vi "Add New Data Channels.vi"(8 "error in (no error)":errorcluster, 11 "Node Ptr":u64 format="%.0x") -> (0 "error out":errorcluster)   [LabVIEW 2019]
uses:
  <vilib>/NI VeriStand/Custom Device API/Custom Device Channel.ctl
  <vilib>/NI VeriStand/Custom Device API/Custom Device Channel Type.ctl
  Shared/Constants.vi
  <vilib>/NI VeriStand/Custom Device API/Set Item Property (String).vi
  <vilib>/NI VeriStand/Custom Device API/Custom Device API.lvlib
  Shared/Instrument Addon Shared.lvlib
panel:
  in  "Tag":string
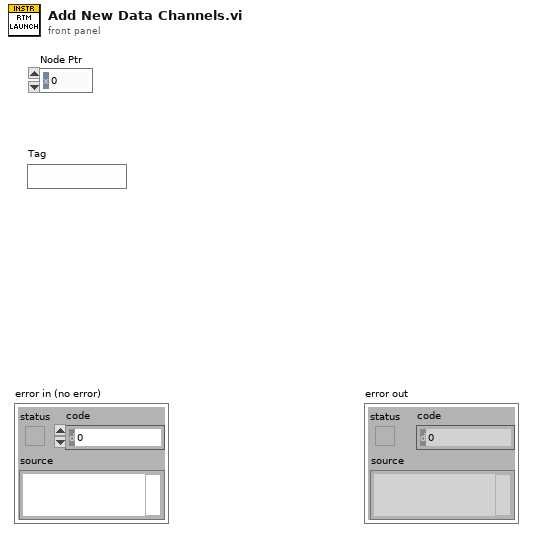
[diagram p1: front panel]
types:
  T1 = typedef "Custom Device API.lvlib/Custom Device Channel.ctl" = cluster{"Type":T2, "Units":string, "Default Value":dbl, "Faultable":bool, "Scalable":bool}
  T2 = typedef "Custom Device API.lvlib/Custom Device Channel Type.ctl" = enum16{"Input", "Output"}
  T3 = typedef "Custom Device API.lvlib/Custom Device Item Ref.ctl" = u64
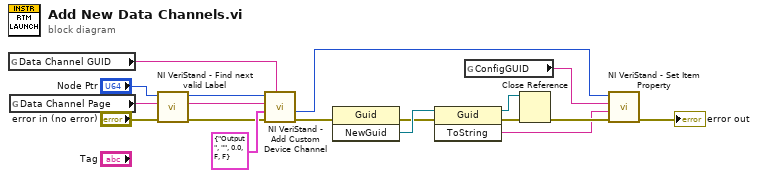
[diagram p0: block diagram]
diagram:
  n1 = global read "Constants.vi" "Data Channel GUID"() -> (w11:string)
  n2 = global read "Constants.vi" "Data Channel Page"() -> (w15:string)
  n3 = call <vilib>:"NI VeriStand - Find next valid Label.vi"("error in (no error)"="error in (no error)", "Label"=w15, "Item Ref in"="Node Ptr") -> ("error out"=w12:errorcluster, "Label out"=w13:string, "Item Ref out"=w14:T3)  [unwired: 4 in, 2 out]
  n4 = call <vilib>:"NI VeriStand - Add Custom Device Channel.vi"("GUID (Default Channel)"=w11, "error in (no error)"=w12, "Channel"=T1 {"Type"=enum."Output", "Units"="", "Default Value"=0.0, "Faultable"=FALSE, "Scalable"=FALSE}, "Channel Name"=w13, "Parent Ref in"=w14) -> ("error out"=w4:errorcluster, "Channel Ref"=w3:T3)  [unwired: 3 in, 2 out]
  n5 = invoke class="Guid" method="NewGuid"(error in=w4) -> (error out=w7:errorcluster, "NewGuid"=w8:refnum<k24>)  [unwired: 2 in, 1 out]
  n6 = invoke class="Guid" method="ToString"(reference=w8, error in=w7) -> (reference out=w9:refnum<k24>, error out=w6:errorcluster, "ToString"=w1:string)  [unwired: 1 in]
  n7 = global read "Constants.vi" "ConfigGUID"() -> (w10:string)
  n8 = Close Reference(reference=w9, error in (no error)=w6) -> (error out=w5:errorcluster)
  n9 = call-poly <vilib>:"NI VeriStand - Set Item Property.vi"("error in (no error)"=w5, "Value"=w1, "Property Name"=w10, "Item Ref in"=w3) -> ("error out"=→"error out":errorcluster)  [unwired: 5 in, 2 out]
